vi "SetupTasks.vi"(9 "eDAQs":T2[][](array[typedef]), 10 "cDAQs":T2[][](array[typedef]), 11 "PXI":T2[][](array[typedef])) -> (0 "cDAQ i":i32[](array[numeric]), 1 "eDAQ i":i32[][](array[numeric]), 2 "cDAQs":refnum<k21>[](array[refnum]), 3 "eDAQs":refnum<k21>[](array[refnum]), 4 "PXI i":i32[][](array[numeric]), 5 "PXIs":refnum<k21>[](array[refnum]), 6 "O PXIs":T1[](array[typedef]))   [LabVIEW 2013]
uses:
  Channels_and_Index.ctl
  AcqControls/Tasks_Indices.ctl
  Globals/Meas_global.vi
  <vilib>/DAQmx/create/channels.llb/DAQmx Create Channel (AI-Voltage-Basic).vi
  <vilib>/regexp/Match Regular Expression.xnode
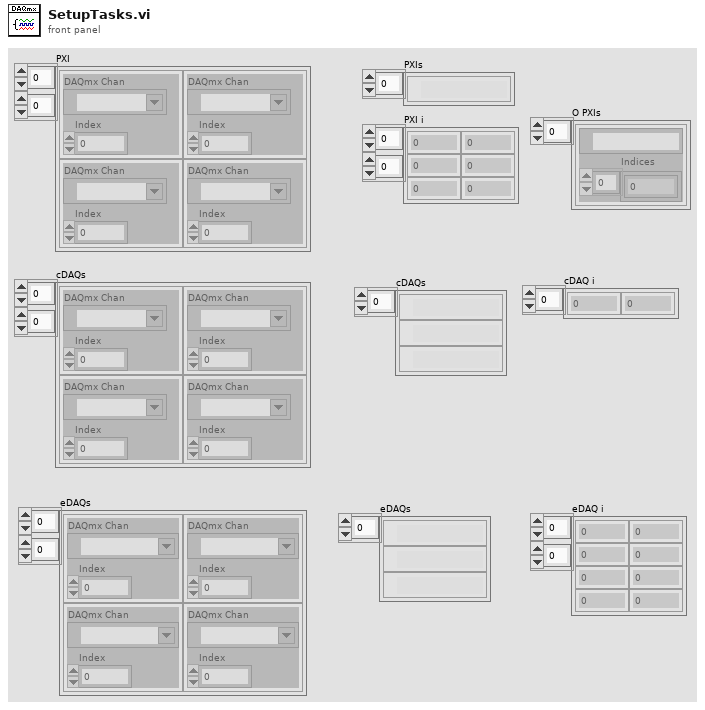
[diagram p1: front panel]
types:
  T1 = typedef "Tasks_Indices.ctl" = cluster{"task out":refnum<k21>, "Indices":i32[]}
  T2 = typedef "Channels_and_Index.ctl" = cluster{"DAQmx Chan":tag, "Index":i32}
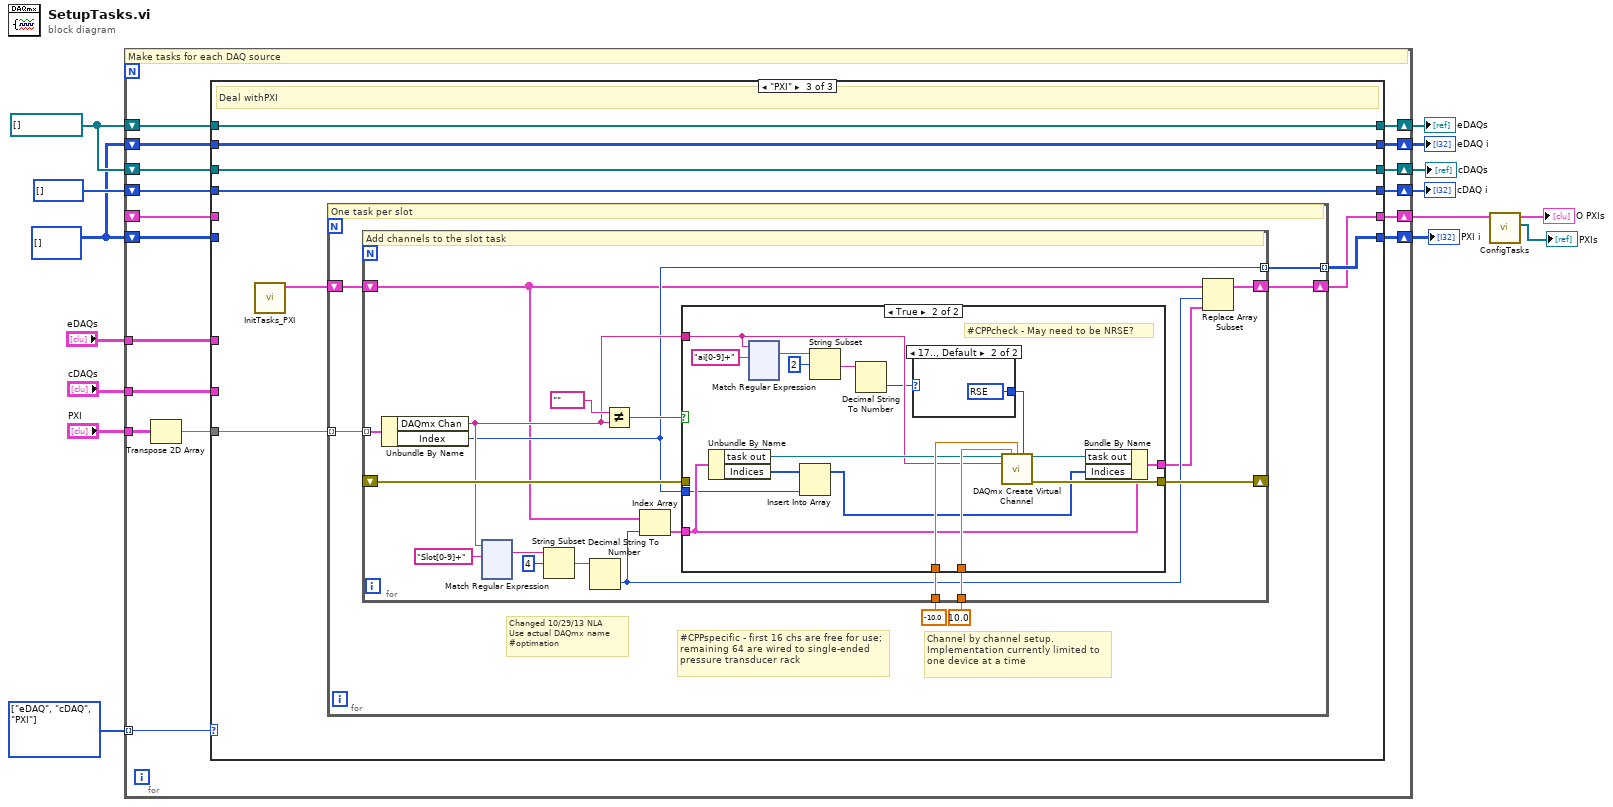
[diagram p0: block diagram]
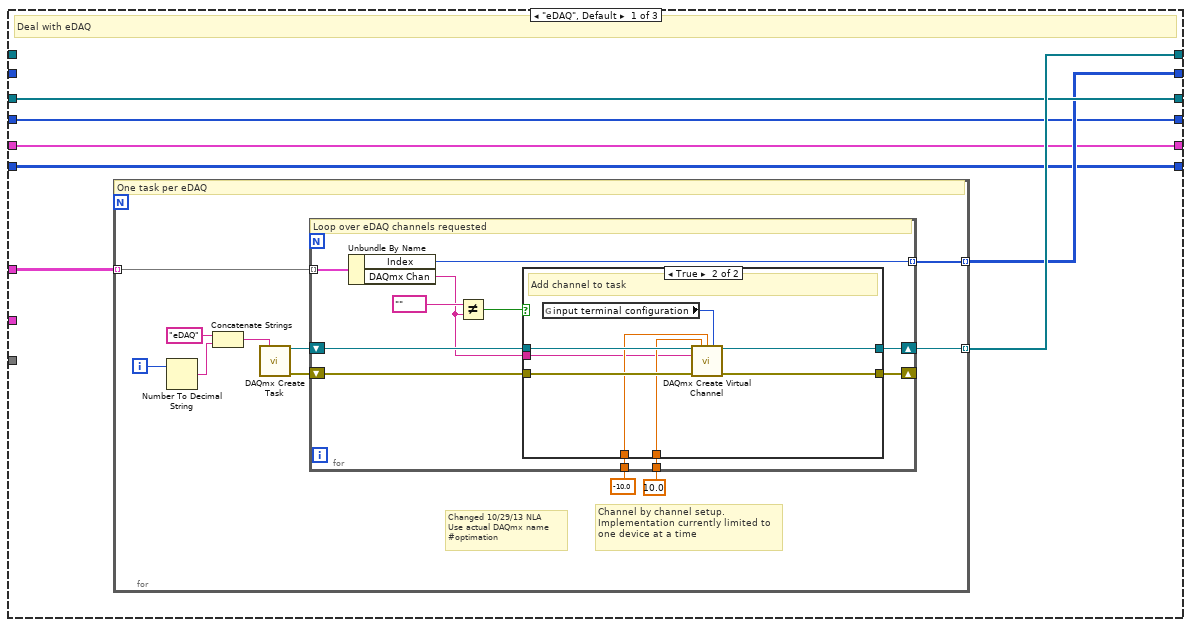
[diagram p2: hidden frame]
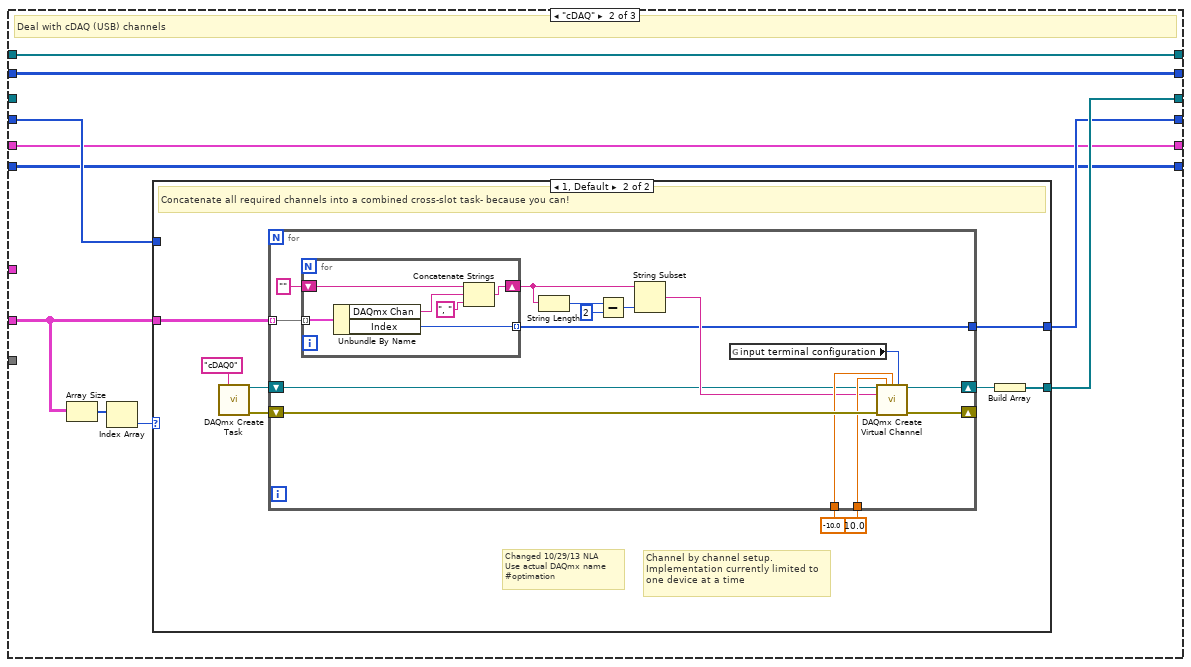
[diagram p4: hidden frame]
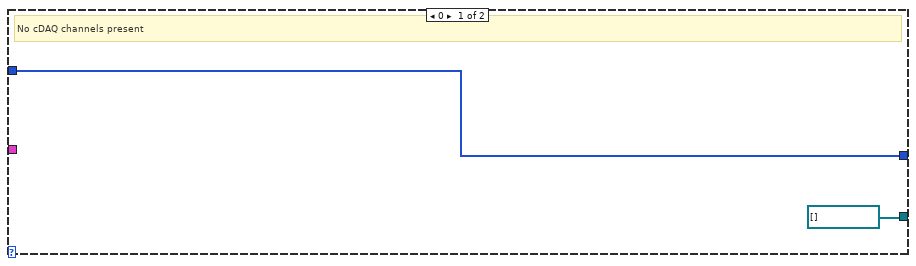
[diagram p5: hidden frame]
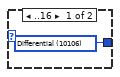
[diagram p7: hidden frame]
diagram:
  w1 = enum16{"eDAQ", "cDAQ", "PXI"}[] [enum."eDAQ", enum."cDAQ", enum."PXI"] items=["eDAQ", "cDAQ", "PXI"]
  w6 = i32[][] []
  w9 = refnum<k21>[] []
  n1 = for {
    tunnel: "eDAQs" -> [w32]
    shift-right: [w31] -> w14
    shift-left: w9 -> [w30]
    tunnel: "cDAQs" -> [w29]
    shift-right: [w28] -> w13
    shift-left: w9 -> [w27]
    shift-right: [w26] -> w10
    shift-left: w6 -> [w25]
    shift-right: [w24] -> w11
    shift-left: i32[] [] -> [w23]
    shift-right: [w20] -> w5
    shift-left: w6 -> [w22]
    tunnel: "PXI" -> [w21]
    shift-right: [w18] -> w4
    shift-left: _ -> [w17]
    tunnel: w1 -> [w16] mode=indexing
    # "Make tasks for each DAQ source"
    n2 = Transpose 2D Array(2D array=w21) -> (transposed array=w19:T2[][])
    n3 = case shown="\"PXI\"" w16 {
      tunnel: w32 -> [w39 _ _]
      tunnel: [w38 w81 w121] -> w31
      tunnel: w30 -> [_ w81 w121]
      tunnel: w29 -> [_ w80 _]
      tunnel: [w37 w78 w118] -> w28
      tunnel: w27 -> [w37 _ w118]
      tunnel: [w36 w77 w120] -> w26
      tunnel: w25 -> [_ w77 w120]
      tunnel: [w35 w76 w117] -> w24
      tunnel: w23 -> [w35 w75 w117]
      tunnel: w22 -> [w34 w74 _]
      tunnel: w19 -> [_ _ w119]
      tunnel: [w34 w74 w116] -> w20
      tunnel: [w33 w73 w114] -> w18
      tunnel: w17 -> [w33 w73 _]
      frame "eDAQ", Default {
        # "Deal with eDAQ"
        n4 = for {
          tunnel: w39 -> [w46] mode=indexing
          tunnel: [w45] -> w38 mode=indexing
          tunnel: [w40] -> w36 mode=indexing
          i -> [w44]
          # "Changed 10/29/13 NLA\nUse actual DAQmx name\n#optimation"
          # "Channel by channel setup. Implementation currently limited to one device at a time"
          # "One task per eDAQ"
          n5 = Number To Decimal String(number=w44) -> (decimal integer string=w43:string)  [unwired: 1 in]
          n6 = Concatenate Strings("eDAQ" ("string"), w43) -> (w41:string)
          n7 = call <vilib>:"DAQmx Create Task.vi"("new task name"=w41) -> ("task out"=w49:refnum<k21>, "error out"=w50:errorcluster)  [unwired: 4 in, 9 out]
          n8 = for {
            shift-right: [w60] -> w45
            shift-left: w49 -> [w61]
            shift-right: [w58] -> _
            shift-left: w50 -> [w59]
            tunnel: -10.0 -> [w57]
            tunnel: 10.0 -> [w56]
            tunnel: w46 -> [w55] mode=indexing
            tunnel: [w51] -> w40 mode=indexing
            # "Loop over eDAQ channels requested"
            n9 = Unbundle By Name(w55) -> ("Index"=w51:i32, "DAQmx Chan"=w52:tag)
            n10 = Not Equal?(x=tag "", y=w52) -> (x != y?=w53:bool)
            n11 = case shown="True" w53 {
              tunnel: w61 -> [w63 w71]
              tunnel: [w63 w70] -> w60
              tunnel: w59 -> [w62 w69]
              tunnel: [w62 w68] -> w58
              tunnel: w57 -> [_ w67]
              tunnel: w56 -> [_ w66]
              tunnel: w52 -> [_ w64]
              frame False {
                # "Channel is a non-channel"
              }
              frame True {
                # "Add channel to task"
                n12 = global read "Meas_global.vi" "input terminal configuration"() -> (w65:i32)
                n13 = call-poly <vilib>:"DAQmx Create Virtual Channel.vi"("task in"=w71, "maximum value"=w66, "minimum value"=w67, "input terminal configuration"=w65, "physical channels"=w64, "error in"=w69) -> ("task out"=w70:refnum<k21>, "error out"=w68:errorcluster)  [unwired: 3 in, 5 out]
              }
            }
          }
        }
      }
      frame "cDAQ" {
        # "Deal with cDAQ (USB) channels"
        n14 = Array Size(array=w80) -> (size(s)=w79:i32[])
        n15 = Index Array(array=w79) -> (element=w72:i32)  [unwired: 1 in]
        n16 = case shown="1, Default" w72 {
          tunnel: w80 -> [_ w92]
          tunnel: [refnum<k21>[] [] w85] -> w78
          tunnel: [w82 w84] -> w76
          tunnel: w75 -> [w82 _]
          frame 0 {
            # "No cDAQ channels present"
          }
          frame 1, Default {
            # "Changed 10/29/13 NLA\nUse actual DAQmx name\n#optimation"
            # "Channel by channel setup. Implementation currently limited to one device at a time"
            # "Concatenate all required channels into a combined cross-slot task- because you can!"
            n17 = call <vilib>:"DAQmx Create Task.vi"("new task name"="cDAQ0") -> ("task out"=w90:refnum<k21>, "error out"=w91:errorcluster)  [unwired: 4 in, 9 out]
            n18 = for {
              shift-right: [w107] -> w87
              shift-left: w90 -> [w95]
              shift-right: [w105] -> _
              shift-left: w91 -> [w106]
              tunnel: -10.0 -> [w104]
              tunnel: 10.0 -> [w103]
              tunnel: w92 -> [w97] mode=indexing
              tunnel: [w94] -> w84
              n19 = for {
                shift-right: [w111] -> w99
                shift-left: "" -> [w110]
                tunnel: w97 -> [w109] mode=indexing
                tunnel: [w108] -> w94 mode=indexing
                n20 = Unbundle By Name(w109) -> ("DAQmx Chan"=w113:tag, "Index"=w108:i32)
                n21 = Concatenate Strings(w110, w113, ", " ("string")) -> (w111:string)
              }
              n22 = String Length(string=w99) -> (length=w101:i32)
              n23 = Subtract(x=w101, y=2) -> (x-y=w100:i32)
              n24 = String Subset(string=w99, length (rest)=w100) -> (substring=w96:string)  [unwired: 1 in]
              n25 = global read "Meas_global.vi" "input terminal configuration"() -> (w93:i32)
              n26 = call-poly <vilib>:"DAQmx Create Virtual Channel.vi"("task in"=w95, "maximum value"=w103, "minimum value"=w104, "input terminal configuration"=w93, "physical channels"=w96, "error in"=w106) -> ("task out"=w107:refnum<k21>, "error out"=w105:errorcluster)  [unwired: 3 in, 5 out]
            }
            n27 = Build Array(w87) -> (w85:refnum<k21>[])
          }
        }
      }
      frame "PXI" {
        # "Deal withPXI"
        n28 = call "InitTasks_PXI.vi"() -> ("PXI_Cluster"=w115:T1[])  [unwired: 11 in]
        n29 = for {
          tunnel: w119 -> [w125] mode=indexing
          tunnel: [w124] -> w116 mode=indexing
          shift-right: [w122] -> w114
          shift-left: w115 -> [w123]
          # "#CPPspecific - first 16 chs are free for use; remaining 64 are wired to single-ended pressure transducer rack"
          # "Changed 10/29/13 NLA\nUse actual DAQmx name\n#optimation"
          # "Channel by channel setup. Implementation currently limited to one device at a time"
          # "One task per slot"
          n30 = for {
            shift-right: [w144] -> _
            shift-left: _ -> [w145]
            tunnel: -10.0 -> [w143]
            tunnel: 10.0 -> [w142]
            tunnel: w125 -> [w141] mode=indexing
            tunnel: [w130] -> w124 mode=indexing
            shift-right: [w128] -> w122
            shift-left: w123 -> [w129]
            # "Add channels to the slot task"
            n31 = Unbundle By Name(w141) -> ("DAQmx Chan"=w136:tag, "Index"=w130:i32)
            n32 = xnode "Match Regular Expression"("input string"=w136, "regular expression"="Slot[0-9]+") -> ("whole match"=w135:string)  [unwired: 4 in, 4 out]
            n33 = String Subset(string=w135, offset (0)=4) -> (substring=w133:string)  [unwired: 1 in]
            n34 = Decimal String To Number(string=w133) -> (number=w132:i32)  [unwired: 2 in, 1 out]
            n35 = Not Equal?(x=tag "", y=w136) -> (x != y?=w139:bool)
            n36 = Index Array(array=w129, index=w132) -> (element=w138:T1)
            n37 = case shown="True" w139 {
              tunnel: w138 -> [w261 w274]
              tunnel: [w261 w272] -> w131
              tunnel: w145 -> [w260 _]
              tunnel: [w260 w278] -> w144
              tunnel: w143 -> [_ w277]
              tunnel: w142 -> [_ w276]
              tunnel: w136 -> [_ w269]
              tunnel: w130 -> [_ w270]
              frame False {
                # "The requested channel is blank."
              }
              frame True {
                # "#CPPcheck - May need to be NRSE?"
                n38 = Unbundle By Name(w274) -> ("task out"=w275:refnum<k21>, "Indices"=w262:i32[])
                n39 = xnode "Match Regular Expression"("input string"=w269, "regular expression"="ai[0-9]+") -> ("whole match"=w267:string)  [unwired: 4 in, 4 out]
                n40 = Insert Into Array(array=w262, new element=w270) -> (w271:i32[])  [unwired: 1 in]
                n41 = String Subset(string=w267, offset (0)=2) -> (substring=w264:string)  [unwired: 1 in]
                n42 = Decimal String To Number(string=w264) -> (number=w265:i32)  [unwired: 2 in, 1 out]
                n43 = case shown="17.., Default" w265 {
                  tunnel: [w393 w394] -> w263
                  frame ..16 {
                    w393 = 10106 items=["default"=-1, "RSE"=10083, "NRSE"=10078, "Differential"=10106, "Pseudodifferential"=12529] ("input terminal configuration")
                  }
                  frame 17.., Default {
                    w394 = 10083 items=["default"=-1, "RSE"=10083, "NRSE"=10078, "Differential"=10106, "Pseudodifferential"=12529] ("input terminal configuration")
                  }
                }
                n44 = call-poly <vilib>:"DAQmx Create Virtual Channel.vi"("task in"=w275, "maximum value"=w276, "minimum value"=w277, "input terminal configuration"=w263, "physical channels"=w269) -> ("task out"=w273:refnum<k21>, "error out"=w278:errorcluster)  [unwired: 4 in, 5 out]
                n45 = Bundle By Name(cluster=w274, "task out"=w273, "Indices"=w271) -> (w272:T1)
              }
            }
            n46 = Replace Array Subset(array=w129, new element=w131, index=w132) -> (w128:T1[])
          }
        }
      }
    }
  }
  "eDAQs" <- w14
  "cDAQs" <- w13
  "cDAQ i" <- w11
  "eDAQ i" <- w10
  "PXI i" <- w5
  n47 = call "ConfigTasks.vi"("Cluster In"=w4) -> ("PXIs"=→"PXIs":refnum<k21>[], "PXI_Cluster"=→"O PXIs":T1[])  [unwired: 9 in]
